vi "AnalysisFetchReults.vi"(8 "error in (no error)":errorcluster, 11 "AnalysisConfig":T6={"PortName"="WLAN_DUT0_ANT0", "PhyPort"=enum."Port5", "ExternalAtt"=0, "TriggerLevel"=-40, "NumberofChain"=1, "AcqLength"=0.0001, "MCSIndex"=7.0, "PhyType"=enum."OFDM", "Standard"=enum."802.11 n", "BW"=enum."20M", "TriggerSource"=enum."RIO0", "Freq"=5180000000.0, "LegacyDataRate"=enum."R1M", "PhyPort2"=enum."Port5", "Freq2"=5180000000.0, "ReferenceLevel(Peak)"=0.0}) -> (0 "error out":errorcluster, 3 "FetchCMD":string[](array[string])=["FETC:RFSA:WLAN:RES:TXP:AVER?", "FETC:RFSA:WLAN:RES:MOD:OFDM:EVM:STR:AVER?", "FETC:RFSA:WLAN:RES:MOD:OFDM:IMP:AVER?", "FETC:RFSA:WLAN:RES:SEM:MARG?"])   [LabVIEW 2015]
uses:
  PhyPort.ctl
  PhyType.ctl
  standard.ctl
  BW.ctl
  LegacyDataRate.ctl
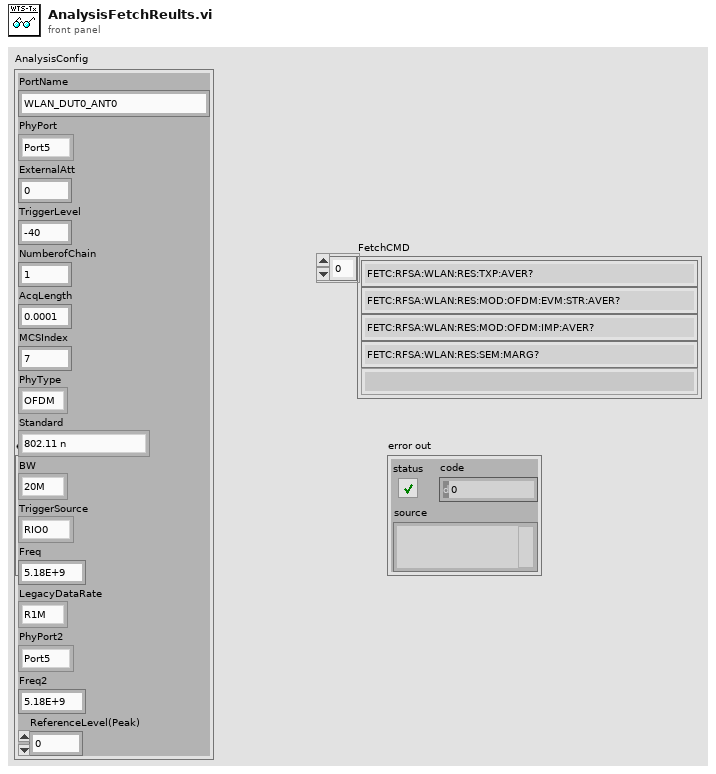
[diagram p1: front panel]
types:
  T1 = typedef "PhyPort.ctl" = enum16{"Port0", "Port1", "Port2", "Port3", "Port4", "Port5", "Port6", "Port7"}
  T2 = typedef "PhyType.ctl" = enum16{"DSSS", "OFDM", "HT", "VHT"}
  T3 = typedef "standard.ctl" = enum16{"802.11 a/g", "802.11 b/g", "802.11 g", "802.11 n", "802.11 ac"}
  T4 = typedef "BW.ctl" = enum16{"5M", "10M", "20M", "40M", "80M", "80P80M", "160M"}
  T5 = typedef "LegacyDataRate.ctl" = enum16{"R1M", "R2M", "R5M5", "R6M", "R9M", "R11M", "R12M", "R18M", "R24M", "R36M", "R48M", "R54M"}
  T6 = cluster{"PortName":string, "PhyPort":T1, "ExternalAtt":i32, "TriggerLevel":i32, "NumberofChain":i32, "AcqLength":dbl, "MCSIndex":dbl, "PhyType":T2, "Standard":T3, "BW":T4, "TriggerSource":enum16{"RIO0", "RIO1"}, "Freq":dbl, "LegacyDataRate":T5, "PhyPort2":T1, "Freq2":dbl, "ReferenceLevel(Peak)":dbl}
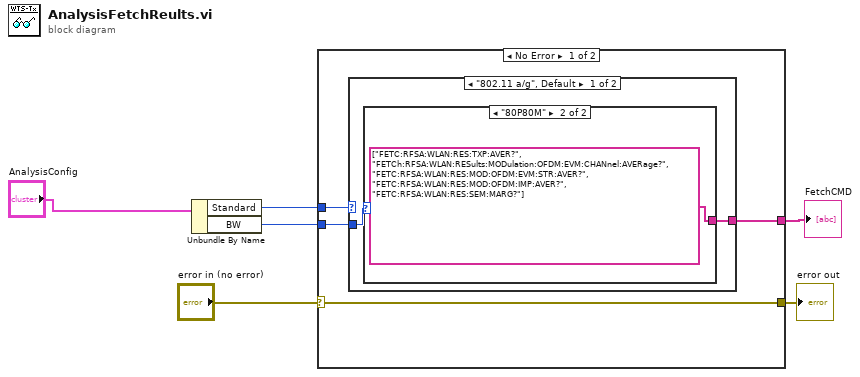
[diagram p0: block diagram]
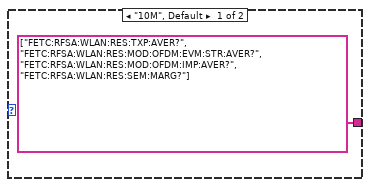
[diagram p2: hidden frame]
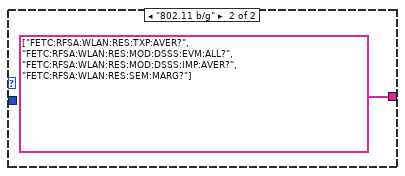
[diagram p3: hidden frame]
diagram:
  n1 = Unbundle By Name("AnalysisConfig") -> ("Standard"=w3:T3, "BW"=w2:T4)
  n2 = case shown="No Error" "error in (no error)" {
    selector: "error in (no error)" -> [w9 w16]
    tunnel: [w10 _] -> w6
    tunnel: [w9 w16] -> w4
    tunnel: w3 -> [w8 _]
    tunnel: w2 -> [w7 _]
    frame No Error {
      n3 = case shown="\"802.11 a/g\", Default" w8 {
        tunnel: [w12 string[] ["FETC:RFSA:WLAN:RES:TXP:AVER?", "FETC:RFSA:WLAN:RES:MOD:DSSS:EVM:ALL?", "FETC:RFSA:WLAN:RES:MOD:DSSS:IMP:AVER?", "FETC:RFSA:WLAN:RES:SEM:MARG?"]] -> w10
        tunnel: w7 -> [w11 _]
        frame "802.11 a/g", Default {
          n4 = case shown="\"80P80M\"" w11 {
            tunnel: [string[] ["FETC:RFSA:WLAN:RES:TXP:AVER?", "FETC:RFSA:WLAN:RES:MOD:OFDM:EVM:STR:AVER?", "FETC:RFSA:WLAN:RES:MOD:OFDM:IMP:AVER?", "FETC:RFSA:WLAN:RES:SEM:MARG?"] string[] ["FETC:RFSA:WLAN:RES:TXP:AVER?", "FETCh:RFSA:WLAN:RESults:MODulation:OFDM:EVM:CHANnel:AVERage?", "FETC:RFSA:WLAN:RES:MOD:OFDM:EVM:STR:AVER?", "FETC:RFSA:WLAN:RES:MOD:OFDM:IMP:AVER?", "FETC:RFSA:WLAN:RES:SEM:MARG?"]] -> w12
            frame "10M", Default {
            }
            frame "80P80M" {
            }
          }
        }
        frame "802.11 b/g" {
        }
      }
    }
    frame Error {
    }
  }
  "error out" <- w4
  "FetchCMD" <- w6
